vi "Prueba1_Albi Jacelyn Cantor.vi"() -> ()   [LabVIEW 2011]
panel:
  out "ALARMA":bool
  out "Temperatura":dbl(slide) scale=0.0..100.0
  out "Velocidad S. RAPIDA":bool
  out "Velocidad RAPIDA":bool
  out "Velocidad lenta":bool
  out "Velocidad":i32(knob) scale=0.0..220.0
  # "SE TIENE QUE GENERAR LA VELOCIDAD ENTRE 1-220 \nLUEGO SE ENCIENDEN LOS LED DE ACUERDO A LA VELOCIDAD\n\n1-80 LENTA\n81-120 RAPIDA\n212-220 MUY RAPIDA\n\nLUEGO SI LA TEMPERATURA ESTA ARRIBA DE LOS 75 GRADOS Y LA VELOCIDAD\nES MUY RAPIDA SE TIENE QUE ENCENDER EL LED DE ALARMA"
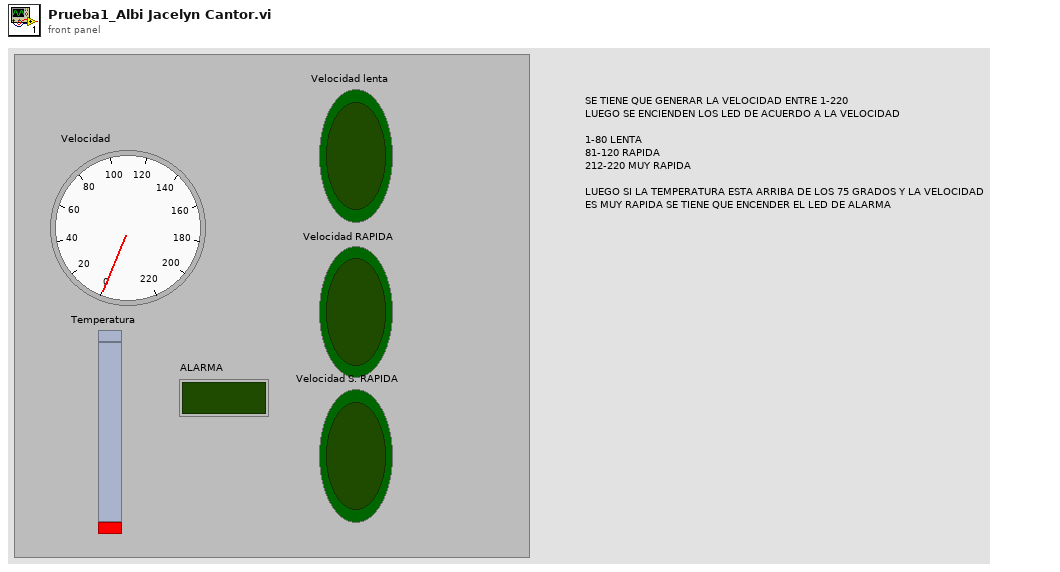
[diagram p1: front panel]
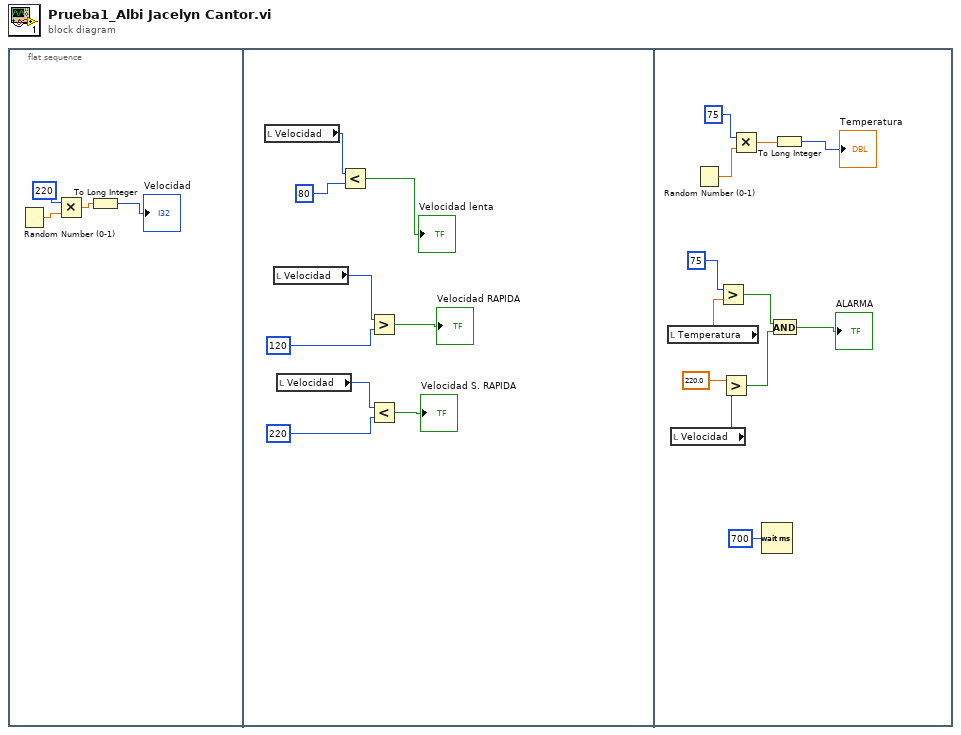
[diagram p0: block diagram]
diagram:
  n1 = flat-sequence {
    frame #0 {
      n2 = Random Number (0-1)() -> (number: 0 to 1=w3:dbl)
      n3 = Multiply(x=220, y=w3) -> (x*y=w2:dbl)
      n4 = To Long Integer(number=w2) -> (32bit integer=→"Velocidad":i32)
    }
    frame #1 {
      n5 = local read "Velocidad"() -> (w7:i32)
      n6 = local read "Velocidad"() -> (w6:i32)
      n7 = local read "Velocidad"() -> (w5:i32)
      n8 = Less?(x=w7, y=80) -> (x < y?=→"Velocidad lenta":bool)
      n9 = Greater?(x=w6, y=120) -> (0:→"Velocidad RAPIDA":bool)
      n10 = Less?(x=w5, y=220) -> (x < y?=→"Velocidad S. RAPIDA":bool)
    }
    frame #2 {
      n11 = local read "Temperatura"() -> (w15:dbl)
      n12 = local read "Velocidad"() -> (w16:i32)
      n13 = Random Number (0-1)() -> (number: 0 to 1=w24:dbl)
      n14 = Greater?(x=75, y=w15) -> (0:w20:bool)
      n15 = Greater?(x=220.0, y=w16) -> (0:w17:bool)
      n16 = Multiply(x=75, y=w24) -> (x*y=w23:dbl)
      n17 = Wait (ms)(milliseconds to wait=u32 700) -> ()  [unwired: 1 out]
      n18 = And(x=w20, y=w17) -> (x .and. y?=→"ALARMA":bool)
      n19 = To Long Integer(number=w23) -> (32bit integer=→"Temperatura":i32)
    }
  }
